vi "SeCrTs-Waveform_Conversion_A.vi"(9 "Irms3":dbl format="%#_13g", 10 "Irms2":dbl format="%#_13g", 11 "Irms1":dbl format="%#_13g") -> (3 "Array":waveform(dbl)[](array[waveform]))   [LabVIEW 2022 SP3]
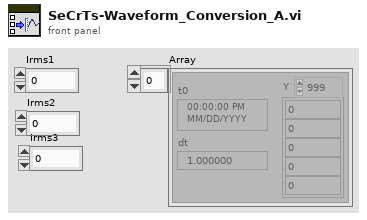
[diagram p1: front panel]
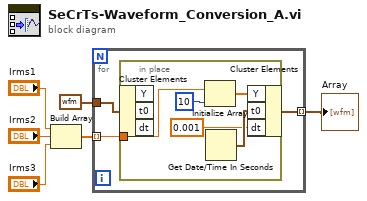
[diagram p0: block diagram]
diagram:
  n1 = Build Array("Irms1", "Irms2", "Irms3") -> (w3:dbl[])
  n2 = for {
    tunnel: w3 -> [w8] mode=indexing
    tunnel: waveform(dbl) {"t0"=timestamp(0 s since 1904-01-01), "dt"=0.001, "Y"=[]} ("waveform") -> [w9]
    tunnel: [w7] -> w1 mode=indexing
    n3 = in-place {
      in-place-border: w8 -> [w12]
      n4 = in-place-cluster #1(w9) -> ()  [unwired: 3 out]
      n5 = Initialize Array(w12, 10 ("dimension size")) -> (w11:dbl[])
      n6 = Get Date/Time In Seconds() -> (seconds since 1Jan1904=w14:timestamp)
      n7 = in-place-cluster #1("Y"=w11, "t0"=w14, "dt"=0.001) -> (w7:waveform(dbl))
    }
  }
  "Array" <- w1
